vi "Processing Step.vi"(8 "error in (no error)":errorcluster, 11 "HTTPStatsHandler in":refnum<class "HTTPStatsHandler.lvclass">) -> (0 "error out":errorcluster, 2 "Step":T1[](array[typedef]), 3 "HTTPStatsHandler out":refnum<class "HTTPStatsHandler.lvclass">)   [LabVIEW 2020, in "Vecto.lvlib" / "HTTPStatsHandler.lvclass"]
uses:
  HTTPStatsHandler.lvclass
  lv-http-server/HTTP Server/Processing Step.ctl
  lv-http-server/HTTP Server/HTTP Server.lvlib
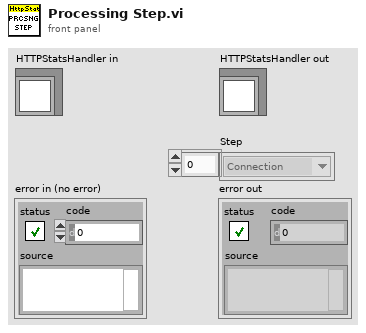
[diagram p1: front panel]
types:
  T1 = typedef "HTTP Server.lvlib/Processing Step.ctl" = enum16{"Connection", "Request", "Routing", "Controller Init", "Controller", "Response", "Complete", "Exception"}
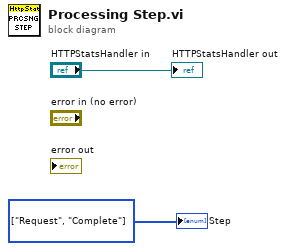
[diagram p0: block diagram]
diagram:
  w1 = T1[] [enum."Request", enum."Complete"] items=["Connection", "Request", "Routing", "Controller Init", "Controller", "Response", "Complete", "Exception"] ("Step")
  "HTTPStatsHandler out" <- "HTTPStatsHandler in"
  "Step" <- w1
